vi "Generate Mock Class.vi"(6 "Add to lvproj?":bool=TRUE, 8 "error in (no error)":errorcluster, 9 "Destination Class Path":path=path "C:/Users/AntonSundqvist/Desktop/New folder/test.lvclass", 10 "Source Class Path":path=path "C:/git/astemes-lmock/tests/Test Doubles/Test Interface/Test Interface.lvclass") -> (0 "error out":errorcluster)   [LabVIEW 2020, in "Mock Class Generator.lvclass"]
uses:
  Mock Class Generator.lvclass
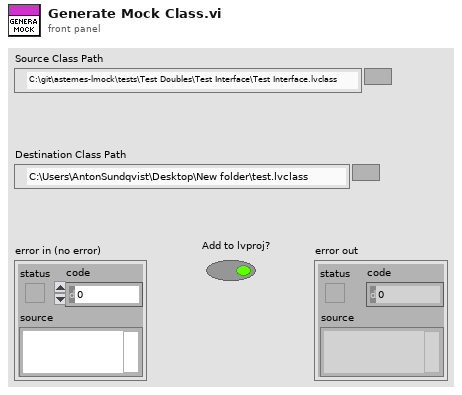
[diagram p1: front panel]
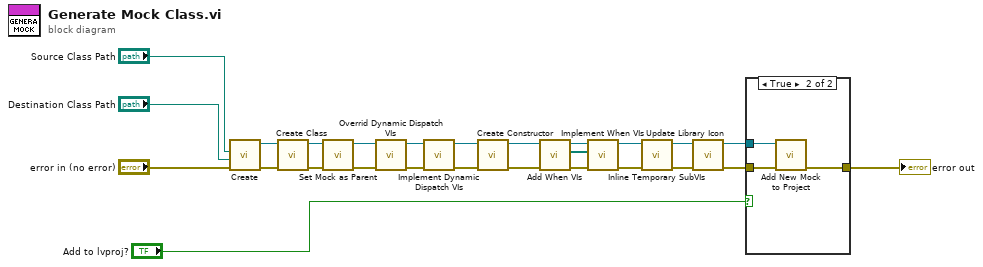
[diagram p0: block diagram]
diagram:
  n1 = call "Create.vi"("error in (no error)"="error in (no error)", "Destination Class Path"="Destination Class Path", "Source Class Path"="Source Class Path") -> ("error out"=w24:errorcluster, "Mock Class Generator Out"=w25:refnum<class "Mock Class Generator.lvclass">)  [unwired: 7 in]
  n2 = call "Create Class.vi"("error in (no error)"=w24, "Mock Class Generator in"=w25) -> ("error out"=w14:errorcluster, "Mock Class Generator out"=w16:refnum<class "Mock Class Generator.lvclass">)  [unwired: 8 in]
  n3 = call "Set Mock as Parent.vi"("error in (no error)"=w14, "Mock Class Generator in"=w16) -> ("error out"=w13:errorcluster, "Mock Class Generator out"=w15:refnum<class "Mock Class Generator.lvclass">)  [unwired: 8 in]
  n4 = call "Overrid Dynamic Dispatch VIs.vi"("error in (no error)"=w13, "Mock Class Generator in"=w15) -> ("error out"=w20:errorcluster, "Mock Class Generator out"=w21:refnum<class "Mock Class Generator.lvclass">)  [unwired: 8 in]
  n5 = call "Implement Dynamic Dispatch VIs.vi"("error in (no error)"=w20, "Mock Class Generator In"=w21) -> ("error out"=w19:errorcluster, "Mock Class Generator Out"=w17:refnum<class "Mock Class Generator.lvclass">)  [unwired: 8 in]
  n6 = call "Create Constructor.vi"("error in (no error)"=w19, "Mock Class Generator in"=w17) -> ("error out"=w11:errorcluster, "Mock Class Generator"=w10:refnum<class "Mock Class Generator.lvclass">)  [unwired: 8 in]
  n7 = call "Add When VIs.vi"("error in (no error)"=w11, "Mock Class Generator In"=w10) -> ("error out"=w9:errorcluster, "When VIs"=w6:path[], "Mock Class Generator Out"=w7:refnum<class "Mock Class Generator.lvclass">)  [unwired: 7 in]
  n8 = call "Implement When VIs.vi"("error in (no error)"=w9, "When VIs"=w6, "Mock Class Generator In"=w7) -> ("error out"=w8:errorcluster, "Mock Class Generator Out"=w4:refnum<class "Mock Class Generator.lvclass">)  [unwired: 7 in]
  n9 = call "Inline Temporary SubVIs.vi"("error in (no error)"=w8, "Responsive Mock Class Generator in"=w4) -> ("error out"=w2:errorcluster, "Responsive Mock Class Generator out"=w1:refnum<class "Mock Class Generator.lvclass">)  [unwired: 8 in]
  n10 = call "Update Library Icon.vi"("error in (no error)"=w2, "Mock Class Generator In"=w1) -> ("error out"=w5:errorcluster, "Mock Class Generator Out"=w3:refnum<class "Mock Class Generator.lvclass">)  [unwired: 8 in]
  n11 = case shown="True" "Add to lvproj?" {
    tunnel: w5 -> [w27 w30]
    tunnel: [w27 w29] -> w18
    tunnel: w3 -> [_ w28]
    frame False {
    }
    frame True {
      n12 = call "Add New Mock to Project.vi"("error in (no error)"=w30, "Mock Class Generator in"=w28) -> ("error out"=w29:errorcluster)  [unwired: 8 in, 1 out]
    }
  }
  "error out" <- w18
